vi "Team and Side.vi"(5 "Lado":enum16{"Esquerdo", "Direito"}(ring) caption="Enum", 7 "Time":enum16{"Azul", "Amarelo"}(ring) caption="Enum", 8 "Goalie":string(combo)="0", 9 "VSS_Ref":T1={"FoulQuadrantVSS"=enum."NO_QUADRANT", "TeamColorVSS"=enum."YELLOW", "HalfVSS"=enum."NO_HALF", "Foul"=enum."FREE_KICK", "timestamp"=0.0}, 10 "Game Status":T19 {"Time" format="%<%.3X %x>T"; "Blue Timeout Remaining" format="%<%M:%S>t"; "Yellow Timeout Remaining" format="%<%M:%S>t"; "Time Left" format="%<%M:%S>t"}, 11 "Field State Input":T2 {"Detection Frame Out"."robots_blue"."height" format="%+4.3f"; "Detection Frame Out"."robots_blue"."pixel_y" format="%+4.3f"; "Detection Frame Out"."robots_blue"."pixel_x" format="%+4.3f"; "Detection Frame Out"."robots_blue"."orientation" format="%+4.3f"; "Detection Frame Out"."robots_blue"."y" format="%+4.3f"; "Detection Frame Out"."robots_blue"."confidence" format="%4.3f"; "Detection Frame Out"."robots_blue"."x" format="%+4.3f"; "Detection Frame Out"."robots_yellow"."height" format="%+4.3f"; "Detection Frame Out"."robots_yellow"."pixel_y" format="%+4.3f"; "Detection Frame Out"."robots_yellow"."pixel_x" format="%+4.3f"; "Detection Frame Out"."robots_yellow"."orientation" format="%+4.3f"; "Detection Frame Out"."robots_yellow"."y" format="%+4.3f"; "Detection Frame Out"."robots_yellow"."confidence" format="%4.3f"; "Detection Frame Out"."robots_yellow"."x" format="%+4.3f"}) -> (1 "VSS_Ref out":T1={"FoulQuadrantVSS"=enum."NO_QUADRANT", "TeamColorVSS"=enum."YELLOW", "HalfVSS"=enum."NO_HALF", "Foul"=enum."FREE_KICK", "timestamp"=0.0}, 3 "IA State":T7={"our_robots"=[], "enemy_robots"=[], "balls"=[], "geometry"={"line_width"=0, "field_length"=0, "field_width"=0, "boundary_width"=0, "referee_width"=0, "goal_width"=0, "goal_depth"=0, "goal_wall_width"=0, "center_circle_radius"=0, "defense_radius"=0, "defense_stretch"=0, "free_kick_from_defense_dist"=0, "penalty_spot_from_field_line_dist"=0, "penalty_line_from_spot_dist"=0}, "IA Judge"={"stage"="", "command"="", "our_goalie_id"=0.0, "enemy_goalie_id"=0.0, "command enum"=enum."Halt", "Time"=enum."Azul"}, "Received Timestamp"=timestamp(0 s since 1904-01-01), "Events"={"Touch"=FALSE, "Ball out"=FALSE, "id touch"=0.0, "Ball out of \nVision"=FALSE, "Ball inside \nGoalie area"=FALSE, "Robot not responding"=FALSE, "Robots responding status"=[1.0, 1.0, 1.0, 1.0, 1.0, 1.0], "Enemy Ball \nPossession"=FALSE, "Pass State"=FALSE, "id end of pass"=0.0, "Kick"=FALSE, "Id ini Possession"=0.0, "Ball Possesion"=FALSE, "Id Possesion"=0.0, "Direct Kick"=FALSE, "2nd Strk Ativo"=FALSE}})   [LabVIEW 2023]
uses:
  SSL Referee Game Status.ctl
  SSL Detection Frame Simple Estimator Cameras VelCmd Folder/Core/AI Input.ctl
  Controls/AI Robot.ctl
  Controls/Functions Enum.ctl
  Controls/AttackerStates.ctl
  Controls/PathDests.ctl
  Controls/PathDest.ctl
  Game_class/Navigation/VSSNavigation/VSSAttackerStates.ctl
  SSL Detection Frame Simple Estimator Cameras VelCmd Folder/Core/AI Ball.ctl
  SSL Detection Frame Simple Estimator Cameras VelCmd Folder/Core/Field Size.ctl
  SSL Detection Frame Simple Estimator Cameras VelCmd Folder/Core/AI Judge.ctl
  Communication_class/Paths/MessageAI_State Folder/Intel/Command Enum.ctl
  SSL Detection Frame Simple Estimator Cameras VelCmd Folder/Util/Events/Events.ctl
  Controls/SSL Field State.ctl
  Controls/SSL Detection Frame.ctl
  Controls/SSL Detection Robot.ctl
  <vilib>/Analysis/Matrix/Datatypes/RealMatrix.ctl
  Controls/SSL Detection Ball.ctl
  Referee_class/VSS_Ref.ctl
  Command.ctl
  <vilib>/Analysis/Matrix/NI_Matrix.lvlib
panel:
  # "Score"
  # "Red Cards"
  # "Yellow Cards"
  # "Timeouts Left"
  # "Timeout Remaining"
  # "Goalie ID"
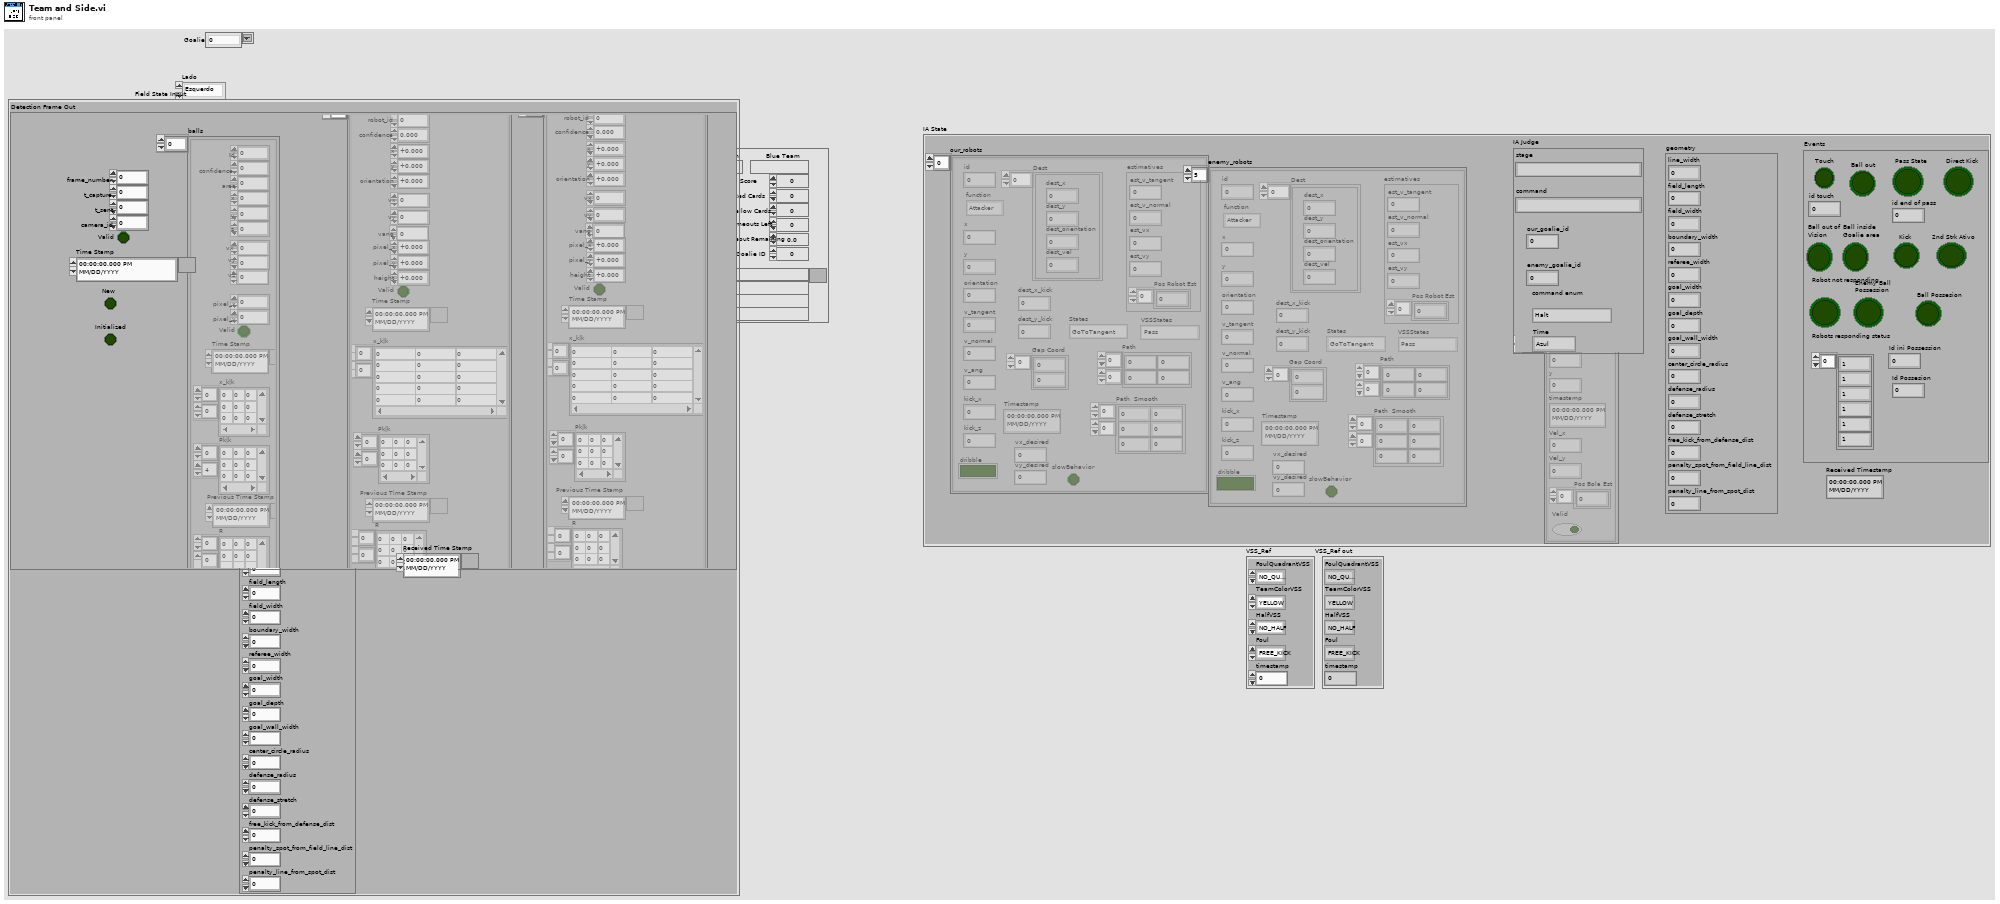
[diagram p1: front panel]
types:
  T1 = typedef "VSS_Ref.ctl" = cluster{"FoulQuadrantVSS":enum16{"NO_QUADRANT", "QUADRANT_1", "QUADRANT_2", "QUADRANT_3", "QUADRANT_4"}, "TeamColorVSS":enum16{"BLUE", "YELLOW", "NONE"}, "HalfVSS":enum16{"NO_HALF", "FIRST_HALF", "SECOND_HALF", "OVERTIME_FIRST_HALF", "OVERTIME_SECOND_HALF", "PENALTY_SHOOTOUS"}, "Foul":enum16{"FREE_KICK", "PENALTY_KICK", "GOAL_KICK", "FREE_BALL", "KICKOFF", "STOP", "GAME_ON", "HALT"}, "timestamp":dbl}
  T2 = typedef "SSL Field State.ctl" = cluster{"Detection Frame Out":T3, "Field Size Out":cluster{"line_width":u32, "field_length":u32, "field_width":u32, "boundary_width":u32, "referee_width":u32, "goal_width":u32, "goal_depth":u32, "goal_wall_width":u32, "center_circle_radius":u32, "defense_radius":u32, "defense_stretch":u32, "free_kick_from_defense_dist":u32, "penalty_spot_from_field_line_dist":u32, "penalty_line_from_spot_dist":u32}, "Received Time Stamp":timestamp}
  T3 = typedef "SSL Detection Frame.ctl" = cluster{"frame_number":u32, "t_capture":dbl, "t_sent":dbl, "camera_id":u32, "robots_yellow":T4[], "robots_blue":T4[], "balls":T6[], "Valid":bool, "Time Stamp":timestamp, "New":bool, "Initialized":bool}
  T4 = typedef "SSL Detection Robot.ctl" = cluster{"x":sgl, "robot_id":u32, "confidence":sgl, "y":sgl, "orientation":sgl, "pixel_x":sgl, "pixel_y":sgl, "height":sgl, "Valid":bool, "Time Stamp":timestamp, "x_k|k":T5, "Pk|k":T5, "Previous Time Stamp":timestamp, "R":T5, "vx":dbl, "vy":dbl, "vang":dbl}
  T5 = typedef "NI_Matrix.lvlib/RealMatrix.ctl" = dbl[][]
  T6 = typedef "SSL Detection Ball.ctl" = cluster{"x":sgl, "area":u32, "confidence":sgl, "y":sgl, "z":sgl, "pixel_x":sgl, "pixel_y":sgl, "Valid":bool, "Time Stamp":timestamp, "x_k|k":T5, "Pk|k":T5, "Id":u32, "Previous Time Stamp":timestamp, "R":T5, " vx":sgl, "vy":dbl, "vz":dbl}
  T7 = typedef "AI Input.ctl" = cluster{"our_robots":T8[], "enemy_robots":T8[], "balls":T14[], "geometry":T15, "IA Judge":T16, "Received Timestamp":timestamp, "Events":T18}
  T8 = typedef "AI Robot.ctl" = cluster{"id":u32, "function":T9, "x":dbl, "y":dbl, "orientation":dbl, "v_tangent":dbl, "v_normal":dbl, "v_ang":dbl, "kick_x":dbl, "kick_z":dbl, "dribble":bool, "Timestamp":timestamp, "estimatives":cluster{"est_v_tangent":dbl, "est_v_normal":dbl, "est_vx":dbl, "est_vy":dbl, "Pos Robot Est":dbl[]}, "dest_x_kick":dbl, "dest_y_kick":dbl, "Gap Coord":dbl[], "States":T10, "Path ":dbl[][], "Path  Smooth":dbl[][], "Dest":T11, "vx_desired":dbl, "vy_desired":dbl, "slowBehavior":bool, "VSSStates":T13}
  T9 = typedef "Functions Enum.ctl" = enum16{"2nd Striker", "Attacker", "Goalie", "Defender", "Striker", "Goto 0", "Dummy", "Kicker", "ZigZag 0", "ZigZag 1", "ZigZag 2", "ZigZag 3", "ZigZag 4", "ZigZag 5", "ZigZag 6", "ZigZag 7", "ZigZag 8", ""}
  T10 = typedef "AttackerStates.ctl" = enum16{"Pass", "GoToTangent", "BallGetting", "GoToKick", ""}
  T11 = typedef "PathDests.ctl" = T12[]
  T12 = typedef "PathDest.ctl" = cluster{"dest_x":dbl, "dest_y":dbl, "dest_orientation":dbl, "dest_vel":dbl}
  T13 = typedef "VSSAttackerStates.ctl" = enum16{"Pass", "GoToTangent", "BallGetting", "GoToKick", "Rotate anti-clockwise", "Rotate Clockwise", ""}
  T14 = typedef "AI Ball.ctl" = cluster{"x":dbl, "y":dbl, "timestamp":timestamp, "Vel_x":dbl, "Vel_y":dbl, "Pos Bola Est":dbl[], "Valid":bool}
  T15 = typedef "Field Size.ctl" = cluster{"line_width":u32, "field_length":u32, "field_width":u32, "boundary_width":u32, "referee_width":u32, "goal_width":u32, "goal_depth":u32, "goal_wall_width":u32, "center_circle_radius":u32, "defense_radius":u32, "defense_stretch":u32, "free_kick_from_defense_dist":u32, "penalty_spot_from_field_line_dist":u32, "penalty_line_from_spot_dist":u32}
  T16 = typedef "AI Judge.ctl" = cluster{"stage":string, "command":string, "our_goalie_id":dbl, "enemy_goalie_id":dbl, "command enum":T17, "Time":enum16{"Azul", "Amarelo"}}
  T17 = typedef "Command Enum.ctl" = enum16{"Halt", "Stop", "Force Start", "PKA Normal Start", "Prepare Kickoff Ally", "PKE Normal Start", "Prepare Kickoff Enemy", "Prepare Penalty Ally", "PPA Normal Start", "Prepare Penalty Enemy", "PPE Normal Start", "Direct Free Enemy", "Direct Free Ally", "Indirect Free Enemy", "Indirect Free Ally", "Timeout Enemy", "Timeout Ally", "Goal Enemy", "Goal Ally", "Ball Placement Enemy", "Ball Placement Ally", "Normal Half Time", "Extra Time Break", "Extra Half Time", "None", "Post Game"}
  T18 = typedef "Events.ctl" = cluster{"Touch":bool, "Ball out":bool, "id touch":dbl, "Ball out of \nVision":bool, "Ball inside \nGoalie area":bool, "Robot not responding":bool, "Robots responding status":dbl[], "Enemy Ball \nPossession":bool, "Pass State":bool, "id end of pass":dbl, "Kick":bool, "Id ini Possession":dbl, "Ball Possesion":bool, "Id Possesion":dbl, "Direct Kick":bool, "2nd Strk Ativo":bool}
  T19 = typedef "SSL Referee Game Status.ctl" = cluster{"Stage":string, "Command":string, "Time Left":dbl, "Yellow Team":string, "Blue Team":string, "Yellow Score":u32, "Blue Score":u32, "Yellow Red Cards":u32, "Blue Red Cards":u32, "Yellow Yellow Cards":u32, "Blue Yellow Cards":u32, "Yellow Timeouts Left":u32, "Blue Timeouts Left":u32, "Yellow Timeout Remaining":dbl, "Blue Timeout Remaining":dbl, "Yellow Goalie Id":u32, "Blue Goalie Id":u32, "Time":timestamp}
  T20 = typedef "Command.ctl" = enum16{"AUTO", "GAME_ON", "STOP", "HALT", "KICKOFF_ALLY", "KICKOFF_ENEMY", "FREE_BALL", "GOAL_KICK_ENEMY", "GOAL_KICK_ALLY", "PENALTY_KICK_ENEMY", "PENALTY_KICK_ALLY", "FREE_KICK"}
  T21 = cluster{"line_width":u32, "field_length":u32, "field_width":u32, "boundary_width":u32, "referee_width":u32, "goal_width":u32, "goal_depth":u32, "goal_wall_width":u32, "center_circle_radius":u32, "defense_radius":u32, "defense_stretch":u32, "free_kick_from_defense_dist":u32, "penalty_spot_from_field_line_dist":u32, "penalty_line_from_spot_dist":u32}
  T22 = enum16{"FREE_KICK", "PENALTY_KICK", "GOAL_KICK", "FREE_BALL", "KICKOFF", "STOP", "GAME_ON", "HALT"}
  T23 = enum16{"NO_QUADRANT", "QUADRANT_1", "QUADRANT_2", "QUADRANT_3", "QUADRANT_4"}
  T24 = enum16{"NO_HALF", "FIRST_HALF", "SECOND_HALF", "OVERTIME_FIRST_HALF", "OVERTIME_SECOND_HALF", "PENALTY_SHOOTOUS"}
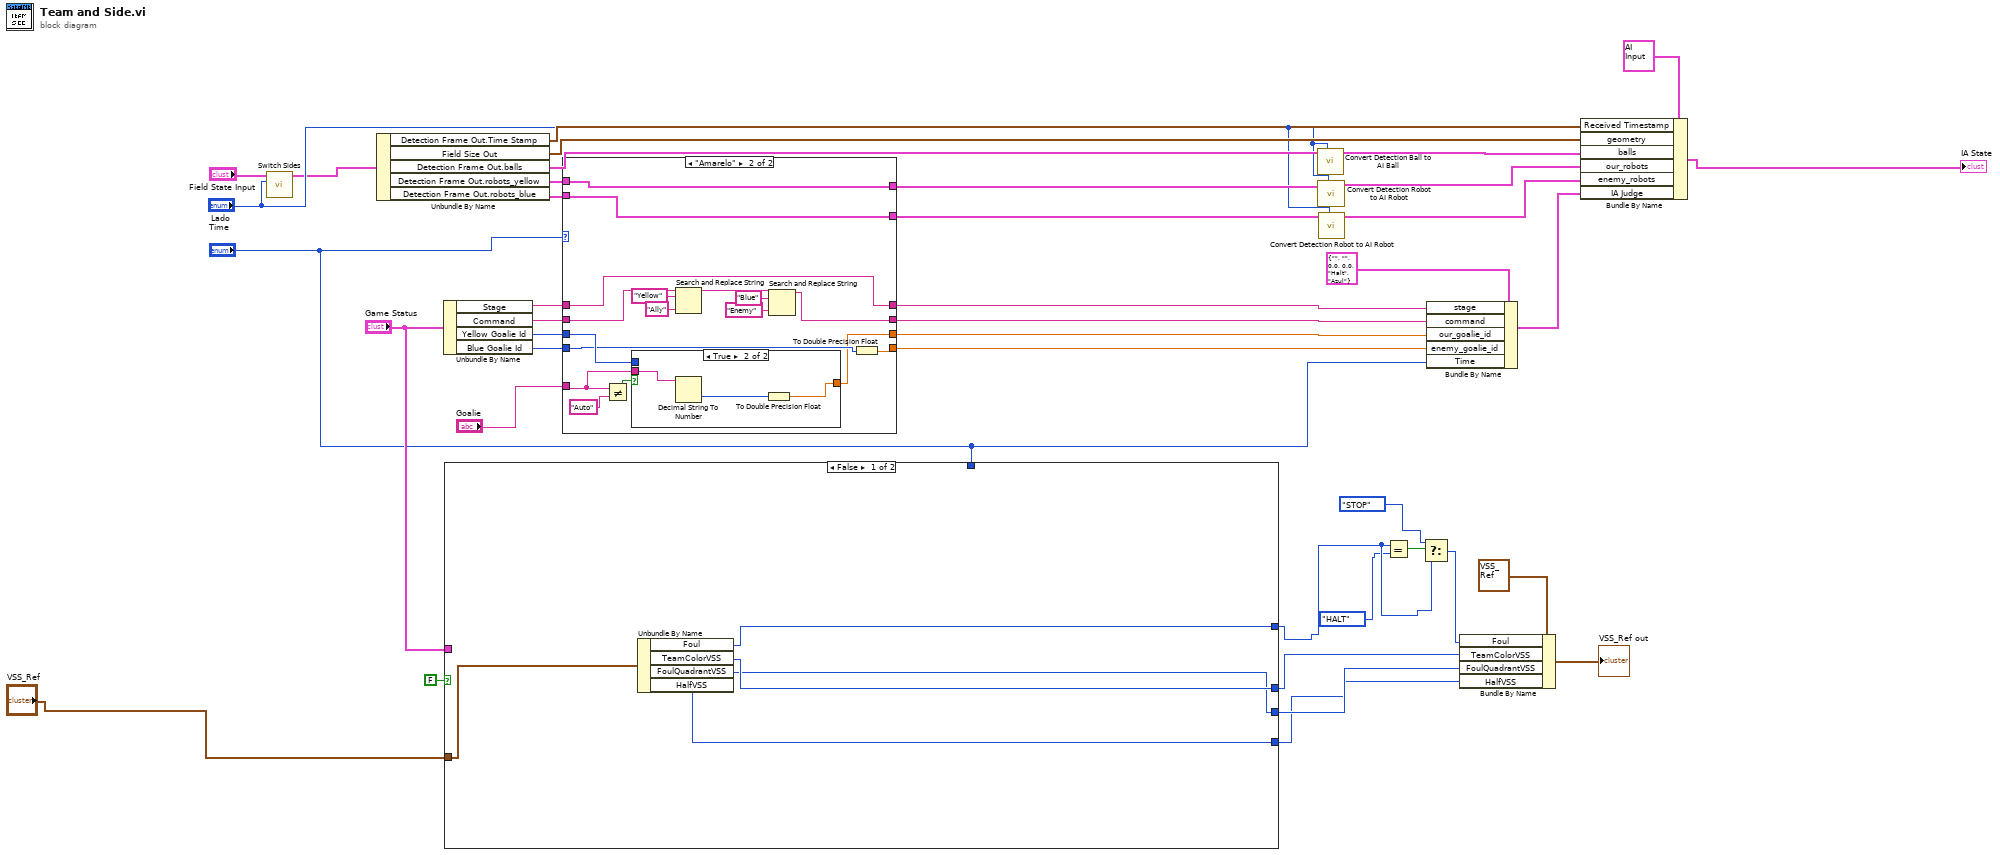
[diagram p0: block diagram]
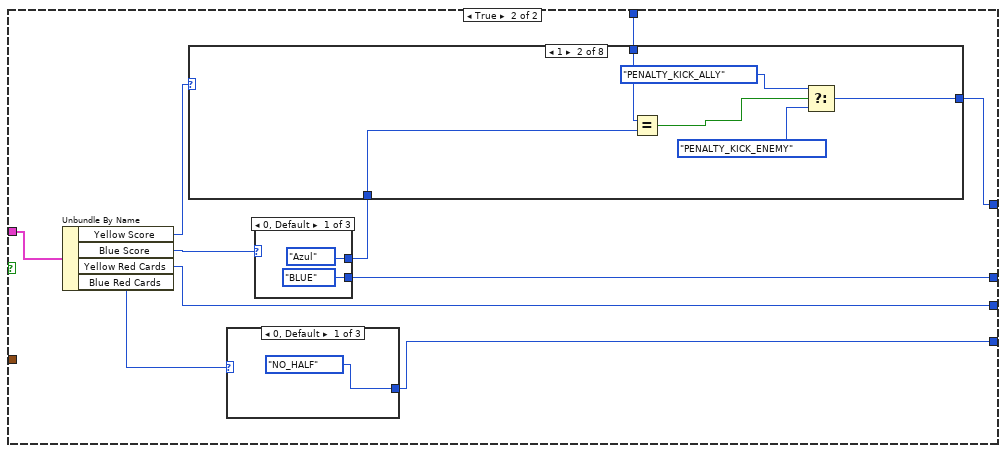
[diagram p2: hidden frame]
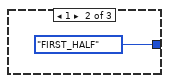
[diagram p3: hidden frame]
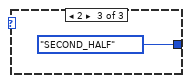
[diagram p4: hidden frame]
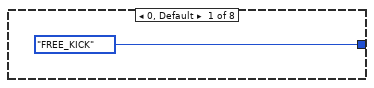
[diagram p5: hidden frame]
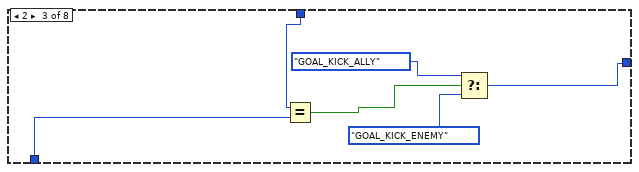
[diagram p6: hidden frame]
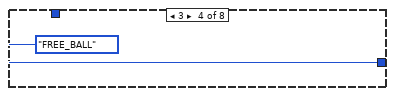
[diagram p7: hidden frame]
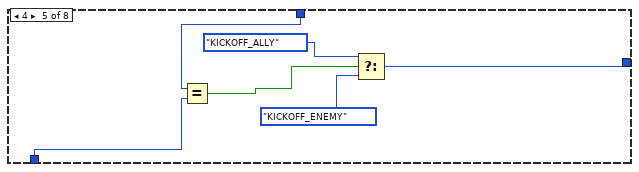
[diagram p8: hidden frame]
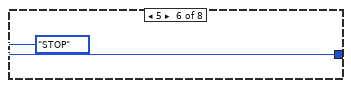
[diagram p9: hidden frame]
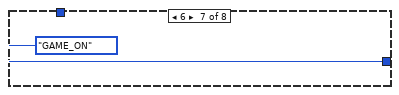
[diagram p10: hidden frame]
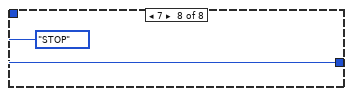
[diagram p11: hidden frame]
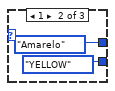
[diagram p12: hidden frame]
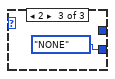
[diagram p13: hidden frame]
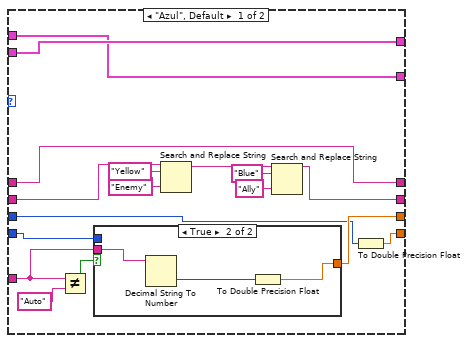
[diagram p14: hidden frame]
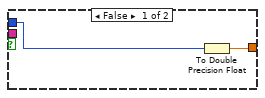
[diagram p15: hidden frame]
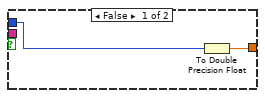
[diagram p16: hidden frame]
diagram:
  n1 = call "Switch Sides.vi"("Lado"="Lado", "Field State Input"="Field State Input") -> ("Field State Side Mirrored"=w18:T2)  [unwired: 9 in]
  n2 = Unbundle By Name(w18) -> ("Detection Frame Out.Time Stamp"=w22:timestamp, "Field Size Out"=w24:T21, "Detection Frame Out.balls"=w25:T6[], "Detection Frame Out.robots_yellow"=w40:T4[], "Detection Frame Out.robots_blue"=w39:T4[])
  n3 = Unbundle By Name("Game Status") -> ("Stage"=w35:string, "Command"=w34:string, "Yellow Goalie Id"=w38:u32, "Blue Goalie Id"=w37:u32)
  n4 = case shown="False" FALSE {
    tunnel: "Game Status" -> [_ w55]
    tunnel: "VSS_Ref" -> [w45 _]
    tunnel: [w41 w48] -> w9
    tunnel: [w43 w52] -> w12
    tunnel: [w42 w50] -> w11
    tunnel: [w44 w49] -> w13
    tunnel: "Time" -> [_ w46]
    frame False {
      n5 = Unbundle By Name(w45) -> ("Foul"=w41:T22, "TeamColorVSS"=w44:enum16{"BLUE", "YELLOW", "NONE"}, "FoulQuadrantVSS"=w43:T23, "HalfVSS"=w42:T24)
    }
    frame True {
      n6 = Unbundle By Name(w55) -> ("Yellow Score"=w53:u32, "Blue Score"=w54:u32, "Yellow Red Cards"=w52:u32, "Blue Red Cards"=w51:u32)
      n7 = case shown="0, Default" w51 {
        tunnel: [enum16{"SECOND_HALF", "FIRST_HALF", "NO_HALF"}."NO_HALF" ("HalfVSS") enum16{"SECOND_HALF", "FIRST_HALF", "NO_HALF"}."FIRST_HALF" ("HalfVSS") enum16{"SECOND_HALF", "FIRST_HALF", "NO_HALF"}."SECOND_HALF" ("HalfVSS")] -> w50
        frame 0, Default {
        }
        frame 1 {
        }
        frame 2 {
        }
      }
      n8 = case shown="0, Default" w54 {
        tunnel: [enum16{"Azul", "Amarelo"}."Azul" ("Time") enum16{"Azul", "Amarelo"}."Amarelo" ("Time") _] -> w47
        tunnel: [enum16{"NONE", "YELLOW", "BLUE"}."BLUE" ("TeamColorVSS") enum16{"NONE", "YELLOW", "BLUE"}."YELLOW" ("TeamColorVSS") enum16{"NONE", "YELLOW", "BLUE"}."NONE" ("TeamColorVSS")] -> w49
        frame 0, Default {
        }
        frame 1 {
        }
        frame 2 {
        }
      }
      n9 = case shown="1" w53 {
        tunnel: [Command."FREE_KICK" ("FoulVSS") w60 w68 Command."FREE_BALL" ("FoulVSS") w75 Command."STOP" ("FoulVSS") Command."GAME_ON" ("FoulVSS") Command."STOP" ("FoulVSS")] -> w48
        tunnel: w47 -> [_ w62 w66 _ w73 _ _ _]
        tunnel: w46 -> [_ w65 w67 _ w74 _ _ _]
        frame 0, Default {
        }
        frame 1 {
          n10 = Equal?(x=w65, y=w62) -> (x = y?=w61:bool)
          n11 = Select(t=Command."PENALTY_KICK_ALLY" ("y"), s=w61, f=Command."PENALTY_KICK_ENEMY") -> (s? t:f=w60:T20)
        }
        frame 2 {
          n12 = Equal?(x=w67, y=w66) -> (x = y?=w69:bool)
          n13 = Select(t=Command."GOAL_KICK_ALLY" ("y"), s=w69, f=Command."GOAL_KICK_ENEMY") -> (s? t:f=w68:T20)
        }
        frame 3 {
        }
        frame 4 {
          n14 = Equal?(x=w74, y=w73) -> (x = y?=w76:bool)
          n15 = Select(t=Command."KICKOFF_ALLY" ("y"), s=w76, f=Command."KICKOFF_ENEMY") -> (s? t:f=w75:T20)
        }
        frame 5 {
        }
        frame 6 {
        }
        frame 7 {
        }
      }
    }
  }
  n16 = case shown="\"Amarelo\"" "Time" {
    tunnel: w40 -> [w102 w124]
    tunnel: w39 -> [w103 w125]
    tunnel: [w103 w124] -> w29
    tunnel: [w102 w125] -> w27
    tunnel: w38 -> [w89 w112]
    tunnel: w37 -> [w87 w110]
    tunnel: [w88 w111] -> w32
    tunnel: [w90 w109] -> w33
    tunnel: w35 -> [w94 w123]
    tunnel: w34 -> [w96 w122]
    tunnel: [w94 w123] -> w31
    tunnel: [w95 w116] -> w30
    tunnel: "Goalie" -> [w91 w113]
    frame "Azul", Default {
      n17 = Not Equal?(x=w91, y="Auto") -> (x != y?=w92:bool)
      n18 = case shown="True" w92 {
        tunnel: w91 -> [_ w108]
        tunnel: [w105 w106] -> w90
        tunnel: w87 -> [w104 _]
        frame False {
          n19 = To Double Precision Float(number=w104) -> (double precision float=w105:dbl)
        }
        frame True {
          n20 = Decimal String To Number(string=w108) -> (number=w107:i32)  [unwired: 2 in, 1 out]
          n21 = To Double Precision Float(number=w107) -> (double precision float=w106:dbl)
        }
      }
      n22 = Search and Replace String(input string=w96, search string="Yellow", replace string="Enemy" ("replace string (\"\")")) -> (result string=w101:string)  [unwired: 5 in, 3 out]
      n23 = Search and Replace String(input string=w101, search string="Blue", replace string="Ally" ("replace string (\"\")")) -> (result string=w95:string)  [unwired: 5 in, 3 out]
      n24 = To Double Precision Float(number=w89) -> (double precision float=w88:dbl)
    }
    frame "Amarelo" {
      n25 = Not Equal?(x=w113, y="Auto") -> (x != y?=w114:bool)
      n26 = case shown="True" w114 {
        tunnel: w113 -> [_ w130]
        tunnel: [w127 w128] -> w109
        tunnel: w112 -> [w126 _]
        frame False {
          n27 = To Double Precision Float(number=w126) -> (double precision float=w127:dbl)
        }
        frame True {
          n28 = Decimal String To Number(string=w130) -> (number=w129:i32)  [unwired: 2 in, 1 out]
          n29 = To Double Precision Float(number=w129) -> (double precision float=w128:dbl)
        }
      }
      n30 = Search and Replace String(input string=w122, search string="Yellow", replace string="Ally" ("replace string (\"\")")) -> (result string=w117:string)  [unwired: 5 in, 3 out]
      n31 = Search and Replace String(input string=w117, search string="Blue", replace string="Enemy" ("replace string (\"\")")) -> (result string=w116:string)  [unwired: 5 in, 3 out]
      n32 = To Double Precision Float(number=w110) -> (double precision float=w111:dbl)
    }
  }
  n33 = call "Convert Detection Ball to AI Ball.vi"("Lado"="Lado", "Input"=w25) -> ("Output"=w21:T14[])  [unwired: 9 in]
  n34 = call "Convert Detection Robot to AI Robot.vi"("Lado"="Lado", "Input"=w29) -> ("Output"=w28:T8[])  [unwired: 9 in]
  n35 = call "Convert Detection Robot to AI Robot.vi"("Lado"="Lado", "Input"=w27) -> ("Output"=w26:T8[])  [unwired: 9 in]
  n36 = Equal?(x=w9, y=Command."HALT" ("FoulVSS")) -> (x = y?=w10:bool)
  n37 = Select(t=Command."STOP" ("FoulVSS"), s=w10, f=w9) -> (s? t:f=w8:u16)
  n38 = Bundle By Name(cluster=T16 {"stage"="", "command"="", "our_goalie_id"=0.0, "enemy_goalie_id"=0.0, "command enum"=enum."Halt", "Time"=enum."Azul"} ("IA Judge"), "stage"=w31, "command"=w30, "our_goalie_id"=w33, "enemy_goalie_id"=w32, "Time"="Time") -> (w20:T16)
  n39 = Bundle By Name(cluster=T1 {"FoulQuadrantVSS"=enum."NO_QUADRANT", "TeamColorVSS"=enum."YELLOW", "HalfVSS"=enum."NO_HALF", "Foul"=enum."FREE_KICK", "timestamp"=0.0} ("VSS_Ref 5"), "Foul"=w8, "TeamColorVSS"=w13, "FoulQuadrantVSS"=w12, "HalfVSS"=w11) -> (→"VSS_Ref out":T1)
  n40 = Bundle By Name(cluster=T7 {"our_robots"=[], "enemy_robots"=[], "balls"=[], "geometry"={"line_width"=0, "field_length"=0, "field_width"=0, "boundary_width"=0, "referee_width"=0, "goal_width"=0, "goal_depth"=0, "goal_wall_width"=0, "center_circle_radius"=0, "defense_radius"=0, "defense_stretch"=0, "free_kick_from_defense_dist"=0, "penalty_spot_from_field_line_dist"=0, "penalty_line_from_spot_dist"=0}, "IA Judge"={"stage"="Normal First Half Pre", "command"="Halt", "our_goalie_id"=0.0, "enemy_goalie_id"=0.0, "command enum"=enum."Halt", "Time"=enum."Azul"}, "Received Timestamp"=timestamp(0 s since 1904-01-01), "Events"={"Touch"=FALSE, "Ball out"=FALSE, "id touch"=0.0, "Ball out of \nVision"=FALSE, "Ball inside \nGoalie area"=FALSE, "Robot not responding"=FALSE, "Robots responding status"=[1.0, 1.0, 1.0, 1.0, 1.0, 1.0], "Enemy Ball \nPossession"=FALSE, "Pass State"=FALSE, "id end of pass"=0.0, "Kick"=FALSE, "Id ini Possession"=0.0, "Ball Possesion"=FALSE, "Id Possesion"=0.0, "Direct Kick"=FALSE, "2nd Strk Ativo"=FALSE}} ("IA State"), "Received Timestamp"=w22, "geometry"=w24, "balls"=w21, "our_robots"=w28, "enemy_robots"=w26, "IA Judge"=w20) -> (→"IA State":T7)
